vi "CREATE SALES QUERY.vi"(0 "What to Search":string, 5 "Search Column Name":string, 7 "Sorting Column Name":string, 9 "Column to Search In":u16, 12 "Date Range":u16(ring) items=["Greater Than", "Less Than", "Between"], 13 "Dates Less Than":string="8/1/2023", 14 "Dates Greater Than":string="8/1/2023") -> (4 "SQL QUERY":string)   [LabVIEW 2019]
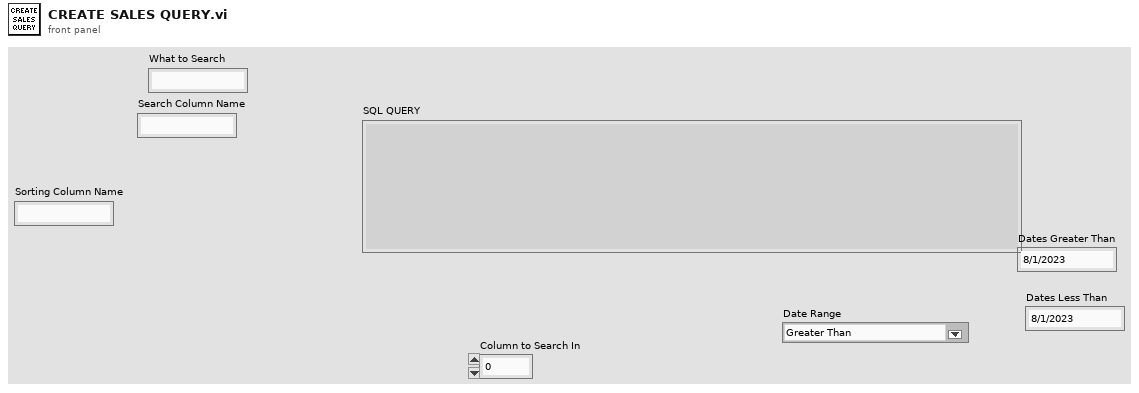
[diagram p1: front panel]
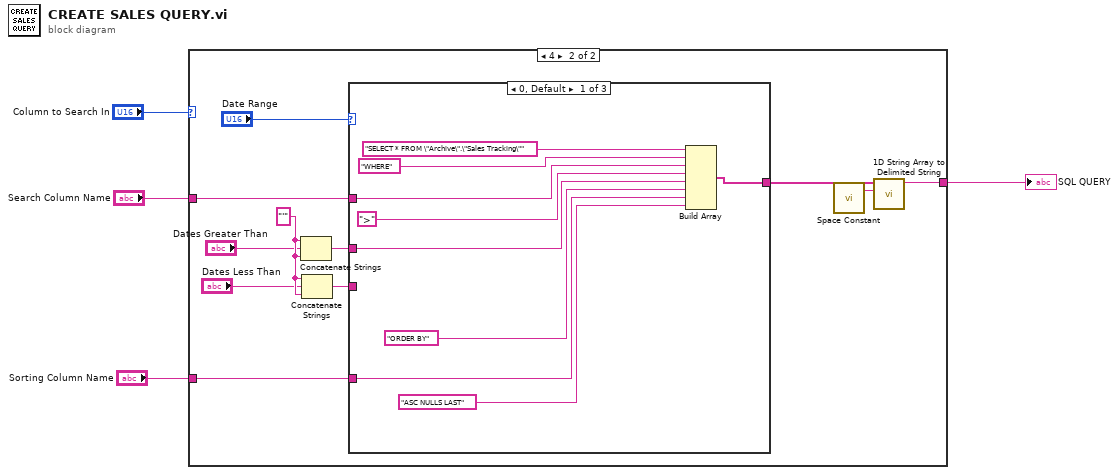
[diagram p0: block diagram]
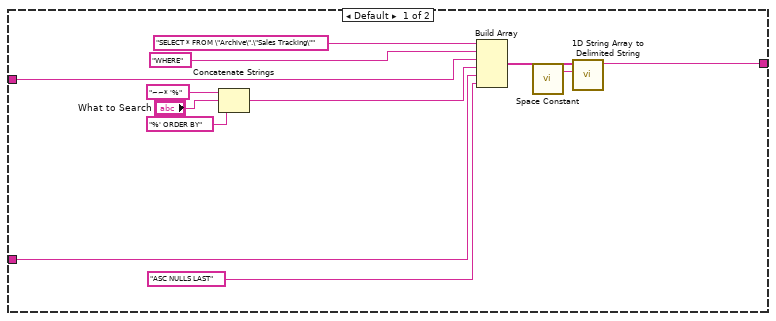
[diagram p2: hidden frame]
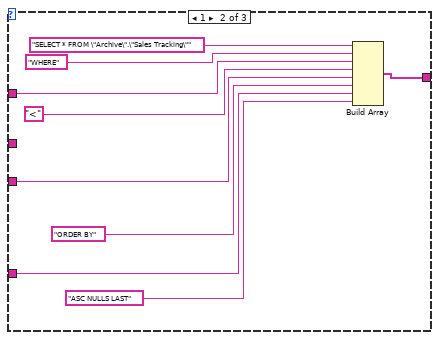
[diagram p3: hidden frame]
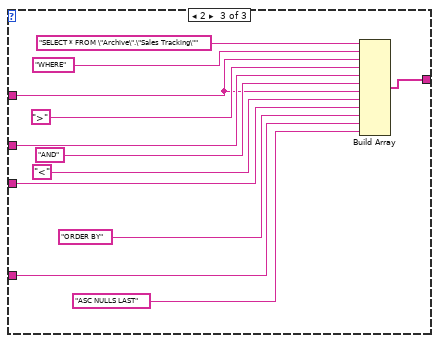
[diagram p4: hidden frame]
diagram:
  n1 = case shown="4" "Column to Search In" {
    tunnel: "Sorting Column Name" -> [w8 w27]
    tunnel: [w5 w26] -> w3
    tunnel: "Search Column Name" -> [w9 w23]
    frame Default {
      n2 = Concatenate Strings("~~* '%" ("string"), "What to Search", "%' ORDER BY" ("string")) -> (w15:string)
      n3 = Build Array("SELECT * FROM \"Archive\".\"Sales Tracking\"" ("string"), "WHERE" ("string"), w9, w15, w8, "ASC NULLS LAST" ("string")) -> (w6:string[])
      n4 = call <vilib>:"Space Constant.vi"() -> ("String"=w7:string)
      n5 = call <vilib>:"1D String Array to Delimited String.vi"("delimiter"=w7, "string array"=w6) -> ("delimited string"=w5:string)  [unwired: 9 in]
    }
    frame 4 {
      w21 = "'"
      n6 = Concatenate Strings(w21, "Dates Greater Than", w21) -> (w18:string)
      n7 = Concatenate Strings(w21, "Dates Less Than", w21) -> (w17:string)
      n8 = case shown="0, Default" "Date Range" {
        tunnel: w27 -> [w28 w37 w46]
        tunnel: [w30 w39 w48] -> w25
        tunnel: w23 -> [w29 w38 w47]
        tunnel: w18 -> [w33 _ w54]
        tunnel: w17 -> [_ w40 w51]
        frame 0, Default {
          n9 = Build Array("SELECT * FROM \"Archive\".\"Sales Tracking\"" ("string"), "WHERE" ("string"), w29, ">" ("string"), w33, "ORDER BY" ("string"), w28, "ASC NULLS LAST" ("string")) -> (w30:string[])
        }
        frame 1 {
          n10 = Build Array("SELECT * FROM \"Archive\".\"Sales Tracking\"" ("string"), "WHERE" ("string"), w38, "<" ("string"), w40, "ORDER BY" ("string"), w37, "ASC NULLS LAST" ("string")) -> (w39:string[])
        }
        frame 2 {
          n11 = Build Array("SELECT * FROM \"Archive\".\"Sales Tracking\"" ("string"), "WHERE" ("string"), w47, ">" ("string"), w54, "AND" ("string"), w47, "<" ("string"), w51, "ORDER BY" ("string"), w46, "ASC NULLS LAST" ("string")) -> (w48:string[])
        }
      }
      n12 = call <vilib>:"Space Constant.vi"() -> ("String"=w24:string)
      n13 = call <vilib>:"1D String Array to Delimited String.vi"("delimiter"=w24, "string array"=w25) -> ("delimited string"=w26:string)  [unwired: 9 in]
    }
  }
  "SQL QUERY" <- w3
